vi "PathToINIBroadcast.vi"(8 "error in (no error)":errorcluster, 10 "PathToINI":path, 11 "ModuleAdmin":refnum<class "ModuleAdmin.lvclass">) -> (0 "error out":errorcluster)   [LabVIEW 2018, in "ScopePlugins.lvlib"]
uses:
  ScopePlugins.lvlib
  <userlib>/NIST/ModuleAdminLib/ModuleAdmin/ModuleAdmin.lvclass
  ScopeShared/clEventType.ctl
  <vilib>/Utility/error.llb/Error Cluster From Error Code.vi
  <vilib>/ErrorRing/Error Ring.xnode
  ScopeShared/ScopeShared.lvlib
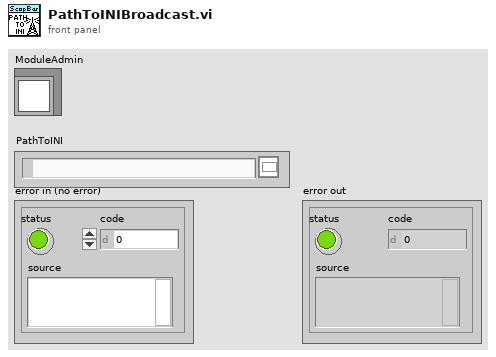
[diagram p1: front panel]
types:
  T1 = typedef "ScopeShared.lvlib/clBroadcastEvents.ctl" = cluster{"DidInit":refnum<user-event>, "StatusUpdate":refnum<user-event>, "ErrorReport":refnum<user-event>, "DidStop":refnum<user-event>, "PathToINI":refnum<user-event>, "Handle":refnum<user-event>, "Model":refnum<user-event>, "Channels":refnum<user-event>, "Acquisition":refnum<user-event>, "Trigger":refnum<user-event>, "ExtAcquisition":refnum<user-event>, "Waveform":refnum<user-event>}
  T2 = typedef "ScopeShared.lvlib/clEventType.ctl" = cluster{"ModuleID":i32, "Data":variant}
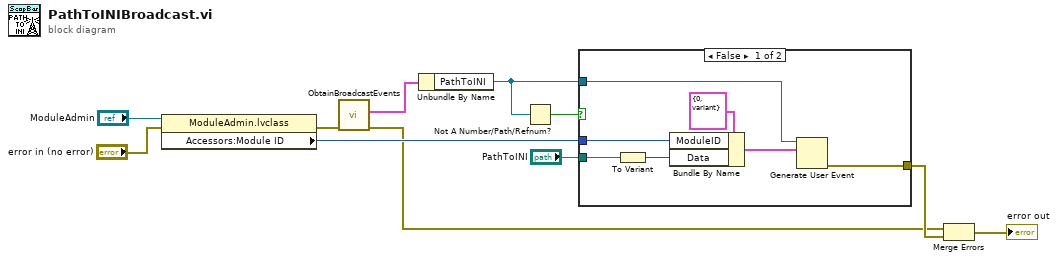
[diagram p0: block diagram]
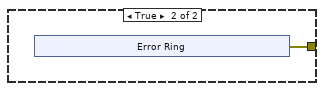
[diagram p2: hidden frame]
diagram:
  n1 = property class="ModuleAdmin.lvclass"(reference="ModuleAdmin", error in="error in (no error)") -> (error out=w2:errorcluster, "Accessors:Module ID"=w3:i32)  [unwired: 1 out]
  n2 = call "ObtainBroadcastEvents.vi"("error in (no error)"=w2) -> ("error out"=w1:errorcluster, "clBroadcastEvents"=w11:T1)  [unwired: 9 in]
  n3 = Unbundle By Name(w11) -> ("PathToINI"=w7:refnum<user-event>)
  n4 = Not A Number/Path/Refnum?(number/path/refnum=w7) -> (NaN/Path/Refnum?=w8:bool)
  n5 = case shown="False" w8 {
    tunnel: w3 -> [w17 _]
    tunnel: "PathToINI" -> [w15 _]
    tunnel: w7 -> [w13 _]
    tunnel: [w12 w19] -> w6
    frame False {
      n6 = To Variant(anything=w15) -> (Variant=w16:variant)
      n7 = Bundle By Name(cluster=T2 {"ModuleID"=0, "Data"=variant} ("clEventType"), "ModuleID"=w17, "Data"=w16) -> (w14:T2)
      n8 = Generate User Event(user event=w13, event data cluster=w14) -> (error out=w12:errorcluster)  [unwired: 2 in, 1 out]
    }
    frame True {
      n9 = xnode "Error Ring"() -> ("error out"=w19:errorcluster)
    }
  }
  n10 = Merge Errors(w1, w6) -> (→"error out":errorcluster)
